vi "F-HomomorphicFilterProcess.vi"() -> ()   [LabVIEW 2014]
doc: "Use this template to build a VI to use as a subVI."
uses:
  <vilib>/vision/NI_Vision_Development_Module.lvlib
panel:
  in  "rh":dbl=60.0
  in  "rl":dbl=128.0
  in  "c":dbl=40.0
  in  "D0":u16=20
  out "|F(u,v)H(u,v)|":T1(plugin-control)
  out "g(x,y)":T1(plugin-control)
  out "IF(u,v)I":T1(plugin-control)
  out "f(x,y)":T1(plugin-control)
  # ":: MVi Framework V1.0 ::\nAuthor:Gaoke Yang\nEmail: gaoke.yang@yahoo.com\nWeb: www.mvicontrol.com\nCopyright (C) 2015, MVI Technologies All Rights Reserved"
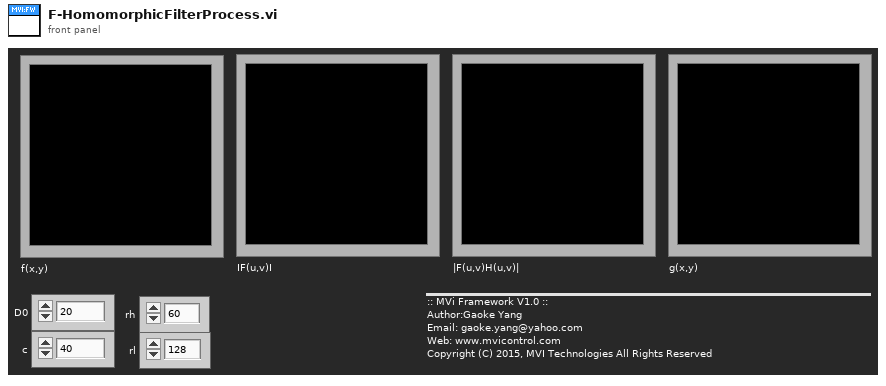
[diagram p1: front panel]
types:
  T1 = typedef "IMAQ Image.ctl" = refnum<image>
  T2 = typedef "Image Type" = u32
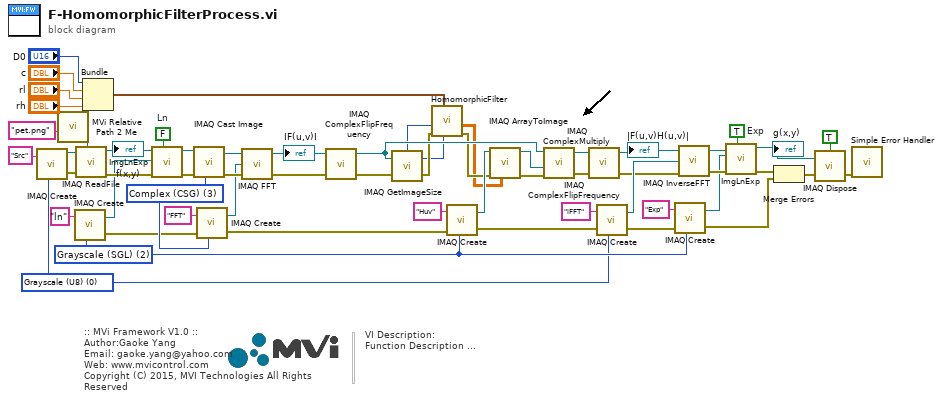
[diagram p0: block diagram]
diagram:
  w1 = T2 0 items=["Grayscale (U8)", "Grayscale (I16)", "Grayscale (SGL)", "Complex (CSG)", "RGB (U32)", "HSL (U32)", "RGB (U64)", "Grayscale (U16)"] ("Image Type")
  w2 = T2 2 items=["Grayscale (U8)", "Grayscale (I16)", "Grayscale (SGL)", "Complex (CSG)", "RGB (U32)", "HSL (U32)", "RGB (U64)", "Grayscale (U16)"] ("Image Type")
  w22 = TRUE  # Exp
  w24 = FALSE  # Ln
  w30 = T2 3 items=["Grayscale (U8)", "Grayscale (I16)", "Grayscale (SGL)", "Complex (CSG)", "RGB (U32)", "HSL (U32)", "RGB (U64)", "Grayscale (U16)"] ("Image Type")
  # "VI Description:\nFunction Description ..."
  # ":: MVi Framework V1.0 ::\nAuthor:Gaoke Yang\nEmail: gaoke.yang@yahoo.com\nWeb: www.mvicontrol.com\nCopyright (C) 2015, MVI Technologies All Rights Reserved"
  n1 = call "IMAQ Create"("Image Name"="Src" ("name or relative path"), "Image Type"=w1) -> ("New Image"=w55:T1, "error out"=w54:errorcluster)  [unwired: 2 in, 1 out]
  n2 = call "MVi Relative Path 2 Me.vi"("Relative Path"="pet.png" ("name or relative path")) -> ("Appended Dir"=w51:path)  [unwired: 5 in, 1 out]
  n3 = call "IMAQ Create"("Image Name"="ln" ("name or relative path"), "Image Type"=w2) -> ("New Image"=w9:T1, "error out"=w10:errorcluster)  [unwired: 2 in, 1 out]
  n4 = call "IMAQ ReadFile"("File Path"=w51, "error in (no error)"=w54, "Image"=w55) -> ("error out"=w25:errorcluster, "Image Out"=w3:T1)  [unwired: 4 in, 3 out]
  "f(x,y)" <- w3
  n5 = Bundle("D0"="D0", "c"="c", "rl"="rl", "rh"="rh") -> (w17:cluster{"D0":u16, "c":dbl, "rl":dbl, "rh":dbl})  [unwired: 1 in]
  n6 = call "ImgLnExp.vi"("Ln/Exp(Ln)"=w24, "EorIn"=w25, "Dst"=w9, "Src"=w3) -> ("ErrOut"=w23:errorcluster, "ImgOut"=w4:T1)  [unwired: 6 in]
  n7 = call "IMAQ Cast Image"("Image Type"=w30, "error in (no error)"=w23, "Image Src"=w4) -> ("error out"=w50:errorcluster, "Image Dst Out"=w48:T1)  [unwired: 7 in]
  n8 = call "IMAQ Create"("Image Name"="FFT" ("name or relative path"), "Image Type"=w30, "error in (no error)"=w10) -> ("New Image"=w47:T1, "error out"=w45:errorcluster)  [unwired: 1 in, 1 out]
  n9 = call "IMAQ FFT"("error in (no error)"=w50, "Image Dst"=w47, "Image Src"=w48) -> ("error out"=w42:errorcluster, "Image Dst Out"=w41:T1)  [unwired: 1 in]
  "IF(u,v)I" <- w41
  n10 = call "IMAQ ComplexFlipFrequency"("error in (no error)"=w42, "Image Src"=w41) -> ("error out"=w36:errorcluster, "Image Dst Out"=w35:T1)  [unwired: 2 in]
  n11 = call "IMAQ GetImageSize"("Image"=w35, "error in (no error)"=w36) -> ("Y Resolution"=w14:i32, "X Resolution"=w16:i32, "error out"=w15:errorcluster)  [unwired: 2 in]
  n12 = call "HomomorphicFilter.vi"("ImgY"=w14, "FilterParam"=w17, "EorIn"=w15, "ImgX"=w16) -> ("ErrOut"=w13:errorcluster, "H(u,v)"=w12:dbl[][])  [unwired: 6 in]
  n13 = call "IMAQ Create"("Image Name"="Huv" ("name or relative path"), "Image Type"=w2, "error in (no error)"=w45) -> ("New Image"=w32:T1, "error out"=w33:errorcluster)  [unwired: 1 in, 1 out]
  n14 = call "IMAQ ArrayToImage"("Image Pixels (Float)"=w12, "error in (no error)"=w13, "Image"=w32) -> ("error out"=w34:errorcluster, "Image Out"=w31:T1)  [unwired: 7 in]
  n15 = call "IMAQ ComplexMultiply"("Image Src A"=w35, "Image Src B"=w31, "error in (no error)"=w34) -> ("Image Dst Out"=w39:T1, "error out"=w40:errorcluster)  [unwired: 4 in]
  n16 = call "IMAQ ComplexFlipFrequency"("error in (no error)"=w40, "Image Src"=w39) -> ("error out"=w38:errorcluster, "Image Dst Out"=w37:T1)  [unwired: 2 in]
  "|F(u,v)H(u,v)|" <- w37
  n17 = call "IMAQ Create"("Image Name"="iFFT" ("name or relative path"), "Image Type"=w1, "error in (no error)"=w33) -> ("New Image"=w43:T1, "error out"=w7:errorcluster)  [unwired: 1 in, 1 out]
  n18 = call "IMAQ Create"("Image Name"="Exp" ("name or relative path"), "Image Type"=w2, "error in (no error)"=w7) -> ("New Image"=w5:T1, "error out"=w6:errorcluster)  [unwired: 1 in, 1 out]
  n19 = call "IMAQ InverseFFT"("error in (no error)"=w38, "Image Dst"=w43, "Image Src"=w37) -> ("error out"=w20:errorcluster, "Image Dst Out"=w19:T1)  [unwired: 1 in]
  n20 = call "ImgLnExp.vi"("Ln/Exp(Ln)"=w22, "EorIn"=w20, "Dst"=w5, "Src"=w19) -> ("ErrOut"=w21:errorcluster, "ImgOut"=w18:T1)  [unwired: 6 in]
  "g(x,y)" <- w18
  n21 = Merge Errors(w21, w6) -> (w49:errorcluster)
  n22 = call "IMAQ Dispose"("All Images? (No)"=TRUE, "Image"=w18, "error in (no error)"=w49) -> ("error out"=w56:errorcluster)  [unwired: 3 out]
  n23 = call <vilib>:"Simple Error Handler.vi"("error in (no error)"=w56) -> ()  [unwired: 1 in, 8 out]
